vi "E3_Case.vi"() -> ()   [LabVIEW 2020]
panel:
  out "String":string
  out "Lleno":bool
  out "Tank":dbl(slide) scale=0.0..100.0
  in  "Numeric":u8
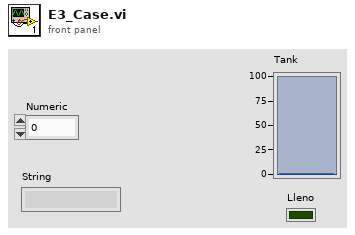
[diagram p1: front panel]
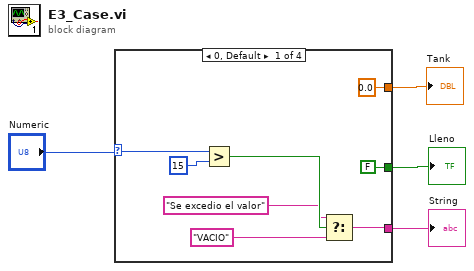
[diagram p0: block diagram]
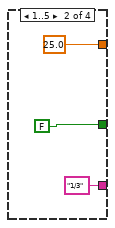
[diagram p2: hidden frame]
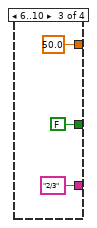
[diagram p3: hidden frame]
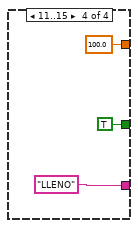
[diagram p4: hidden frame]
diagram:
  n1 = case shown="0, Default" "Numeric" {
    selector: "Numeric" -> [w9 _ _ _]
    tunnel: [0.0 ("Tank") 25.0 ("Tank") 50.0 ("Tank") 100.0 ("Tank")] -> w4
    tunnel: [FALSE ("Lleno") FALSE ("Lleno") FALSE ("Lleno") TRUE ("Lleno")] -> w3
    tunnel: [w10 "1/3" ("String") "2/3" ("String") "LLENO" ("String")] -> w2
    frame 0, Default {
      n2 = Greater?(x=w9, y=u8 15) -> (0:w7:bool)
      n3 = Select(t="Se excedio el valor" ("String"), s=w7, f="VACIO" ("String")) -> (s? t:f=w10:string)
    }
    frame 1..5 {
    }
    frame 6..10 {
    }
    frame 11..15 {
    }
  }
  "Tank" <- w4
  "Lleno" <- w3
  "String" <- w2
